vi "Service Init.vi"(8 "error in (no error)":errorcluster, 9 "NIVS.Workspace Event":refnum<event-registration>, 10 "NIVS.Project File Path":path, 11 "NIVS.Gateway IP Address":string) -> (0 "error out":errorcluster, 3 "System Refs Cluster":T1)   [LabVIEW 2010, in "TDMS to ASCII Convert.lvlib"]
uses:
  TDMS to ASCII Convert.lvlib
  Service Ref Cluster.ctl
  Queue Typedef.ctl
  <vilib>/NI Veristand/Execution/Workspace/WorkspaceAPI.ctl
  NationalInstruments.VeriStand.ClientAPI
  <vilib>/NI Veristand/Execution/Stimulus/StimulusAPI.ctl
  <vilib>/NI Veristand/Execution/Workspace/SystemStateRegEventRef.ctl
  <vilib>/NI Veristand/Execution/Workspace/SystemStateEventRef.ctl
  Stop FGV Commands.ctl
  <vilib>/NI Veristand/Execution/Workspace/NI_VS Workspace ExecutionAPI.lvlib
  <vilib>/NI Veristand/Execution/Stimulus/NI_VS Stimulus ExecutionAPI.lvlib
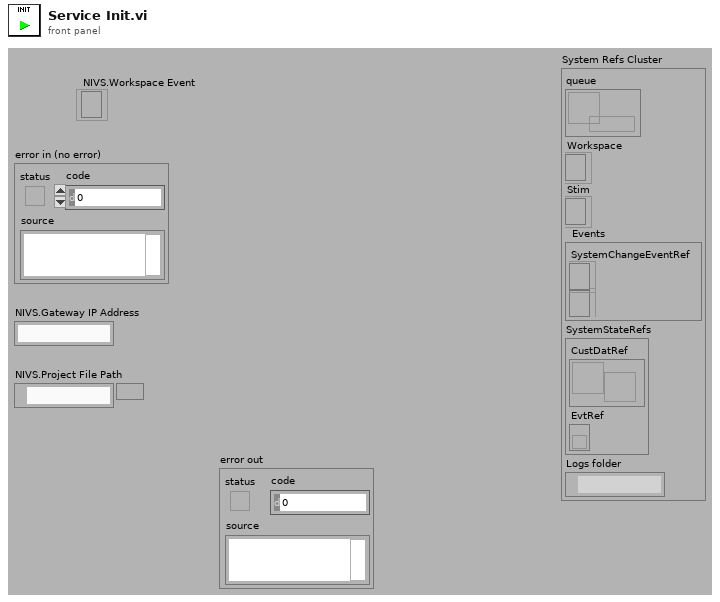
[diagram p1: front panel]
types:
  T1 = typedef "TDMS to ASCII Convert.lvlib/Service Ref Cluster.ctl" = cluster{"queue":refnum<queue>, "Workspace":T2, "Stim":T3, "Events":cluster{"SystemChangeEventRef":T4, "NIVS.Workspace Event":refnum<event-registration>}, "SystemStateRefs":T5, "Logs folder":path}
  T2 = typedef "NI_VS Workspace ExecutionAPI.lvlib/WorkspaceAPI.ctl" = refnum<k24>
  T3 = typedef "NI_VS Stimulus ExecutionAPI.lvlib/StimulusAPI.ctl" = refnum<k24>
  T4 = typedef "NI_VS Workspace ExecutionAPI.lvlib/SystemStateRegEventRef.ctl" = refnum<event-registration>
  T5 = typedef "NI_VS Workspace ExecutionAPI.lvlib/SystemStateEventRef.ctl" = cluster{"CustDatRef":refnum<user-event>, "EvtRef":refnum<k27>}
  T6 = typedef "TDMS to ASCII Convert.lvlib/Queue Typedef.ctl" = cluster{"Path":path, "TDMS Logs":path[]}
  T7 = typedef "TDMS to ASCII Convert.lvlib/Stop FGV Commands.ctl" = enum16{"Write", "Read", "Reset"}
  T8 = cluster{"SystemChangeEventRef":T4, "NIVS.Workspace Event":refnum<event-registration>}
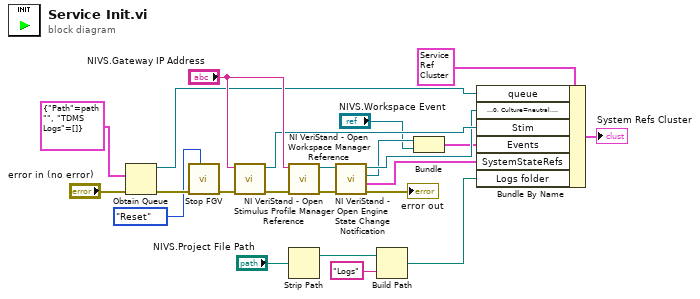
[diagram p0: block diagram]
diagram:
  n1 = Obtain Queue(element data type=T6 {"Path"=path "", "TDMS Logs"=[]} ("Queue Data"), error in (no error)="error in (no error)") -> (queue out=w8:refnum<queue>, error out=w23:errorcluster)  [unwired: 3 in, 1 out]
  n2 = call "Stop FGV.vi"("Command"=Stop_FGV_Commands."Reset", "error in (no error)"=w23) -> ("error out"=w21:errorcluster)  [unwired: 7 in, 2 out]
  n3 = call <vilib>:"NI VeriStand - Open Stimulus Profile Manager Reference.vi"("error in (no error)"=w21, "Gateway IP Address (\"\": localhost)"="NIVS.Gateway IP Address") -> ("error out"=w15:errorcluster, "StimulusProfileManager"=w13:T3)  [unwired: 8 in]
  n4 = call <vilib>:"NI VeriStand - Open Workspace Manager Reference.vi"("error in (no error)"=w15, "Gateway IP Address (\"\": localhost)"="NIVS.Gateway IP Address") -> ("error out"=w3:errorcluster, "WorkspaceManager"=w2:T2)  [unwired: 8 in]
  n5 = Strip Path(path="NIVS.Project File Path") -> (stripped path=w17:path)  [unwired: 1 out]
  n6 = call <vilib>:"NI VeriStand - Open Engine State Change Notification.vi"("error in (no error)"=w3, "WorkspaceManager in"=w2) -> ("error out"=→"error out":errorcluster, "SystemStateRefs"=w12:T5, "SystemChangeEventRef"=w6:T4, "WorkspaceManager out"=w7:T2)  [unwired: 6 in]
  n7 = Build Path(base path=w17, name or relative path="Logs") -> (appended path=w11:path)
  n8 = Bundle("SystemChangeEventRef"=w6, "NIVS.Workspace Event"="NIVS.Workspace Event") -> (w4:T8)  [unwired: 1 in]
  n9 = Bundle By Name(cluster=T1 {"queue"=refnum, "Workspace"=refnum, "Stim"=refnum, "Events"={"SystemChangeEventRef"=refnum, "NIVS.Workspace Event"=refnum}, "SystemStateRefs"={"CustDatRef"=refnum, "EvtRef"=refnum}, "Logs folder"=path ""} ("Service Refs Cluster"), "queue"=w8, "Workspace"=w7, "Stim"=w13, "Events"=w4, "SystemStateRefs"=w12, "Logs folder"=w11) -> (→"System Refs Cluster":T1)
